vi "ExecuteXML.vi"(8 "error in (no error)":errorcluster, 11 "Auto File Path":path=path "C:/Users/Bendethic/Desktop/AutoRoutineCreator/AutoFiles/1A.txt") -> (0 "error out":errorcluster)   [LabVIEW 2017]
panel:
  out "XML String":string
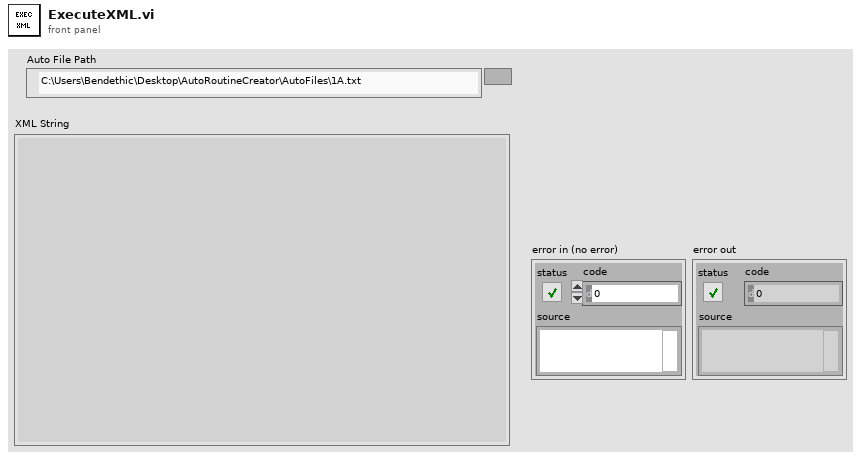
[diagram p1: front panel]
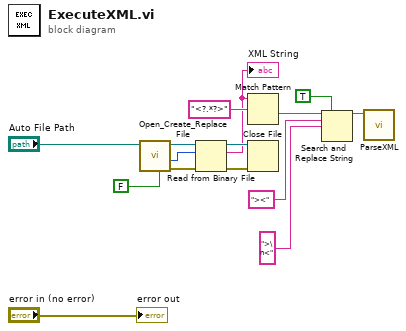
[diagram p0: block diagram]
diagram:
  n1 = call <vilib>:"Open_Create_Replace File.vi"("advisory dialog? (display:T)"=FALSE, "file path"="Auto File Path") -> ("error out"=w12:errorcluster, "file size (bytes)"=w14:i32, "refnum"=w10:refnum<file>)  [unwired: 6 in, 1 out]
  n2 = Read from Binary File(8:w12, 10:w14, 11:w10) -> (0:w13:errorcluster, 2:w8:string, 3:w11:refnum<file>)  [unwired: 3 in, 1 out]
  "XML String" <- w8
  n3 = Match Pattern(string=w8, regular expression="<?.*?>") -> (after substring=w5:string)  [unwired: 1 in, 3 out]
  n4 = Close File(refnum=w11, error in=w13) -> ()  [unwired: 2 out]
  n5 = Search and Replace String(replace all?=TRUE ("replace all? (F)"), input string=w5, search string="><", replace string=">\n<" ("replace string (\"\")")) -> (result string=w2:string)  [unwired: 4 in, 3 out]
  n6 = call "ParseXML.vi"("Node"=w2) -> ()  [unwired: 10 in, 1 out]
  "error out" <- "error in (no error)"
